vi "Calculate Pressure Drop Rate.vi"(2 "Drop Rate Param":T1={"Drop Rate Calc Interval (sec)"=15.0, "Last Pressure (psi)"=0.0, "Allowable Press. Drop/min"=0.0, "Pressure Drop Accepted?"=FALSE, "Block interval to test"=10, "Block counter"=0}, 3 "Current Pressure (psi)":sgl format="%.1f") -> (0 "Drop rate within range?":bool, 1 "Pressure drop rate":dbl)   [LabVIEW 2020]
uses:
  Control/Drop Rate Param.ctl
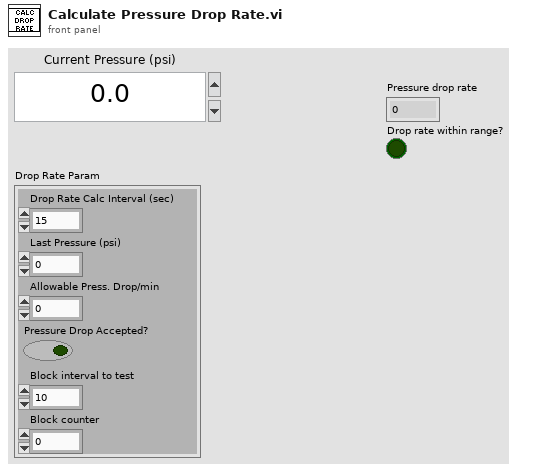
[diagram p1: front panel]
types:
  T1 = typedef "Drop Rate Param.ctl" = cluster{"Drop Rate Calc Interval (sec)":dbl, "Last Pressure (psi)":dbl, "Allowable Press. Drop/min":dbl, "Pressure Drop Accepted?":bool, "Block interval to test":i32, "Block counter":i32}
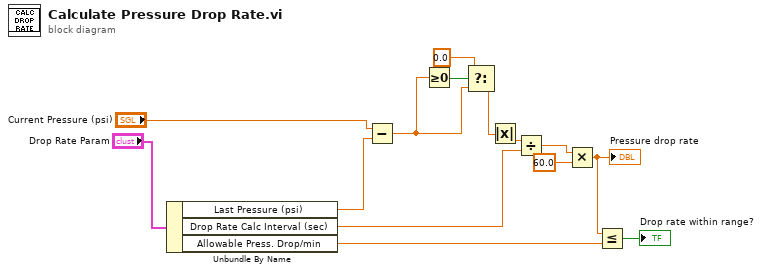
[diagram p0: block diagram]
diagram:
  n1 = Unbundle By Name("Drop Rate Param") -> ("Last Pressure (psi)"=w8:dbl, "Drop Rate Calc Interval (sec)"=w9:dbl, "Allowable Press. Drop/min"=w6:dbl)
  n2 = Subtract(x="Current Pressure (psi)", y=w8) -> (x-y=w3:dbl)
  n3 = Greater Or Equal To 0?(x=w3) -> (x >= 0?=w4:bool)
  n4 = Select(t=0.0, s=w4, f=w3) -> (s? t:f=w1:dbl)
  n5 = Absolute Value(x=w1) -> (abs(x)=w12:dbl)
  n6 = Divide(x=w12, y=w9) -> (x/y=w14:dbl)
  n7 = Multiply(x=w14, y=60.0) -> (x*y=w7:dbl)
  "Pressure drop rate" <- w7
  n8 = Less Or Equal?(x=w7, y=w6) -> (x <= y?=→"Drop rate within range?":bool)
